vi "get parameters.vi"(8 "error in (no error)":errorcluster, 11 "Task.lvclass in":refnum<class "Task.lvclass">) -> (0 "error out":errorcluster, 2 "parameters":T1, 3 "Task.lvclass out":refnum<class "Task.lvclass">)   [LabVIEW 2020, in "Tasks.lvlib" / "Task.lvclass"]
uses:
  Task.lvclass
  parameters.ctl
  Task.lvclass/Task.ctl
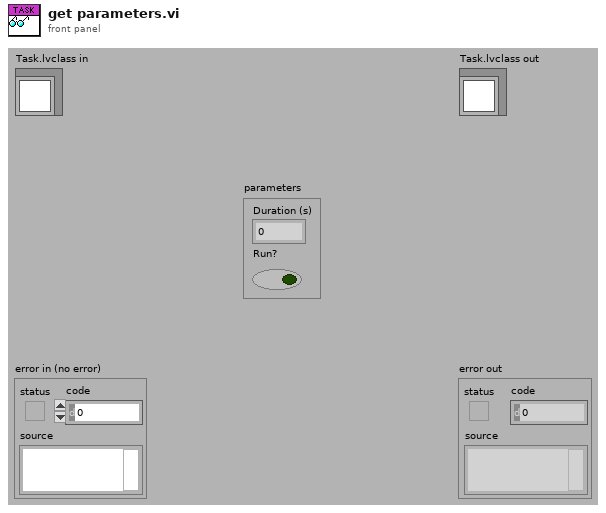
[diagram p1: front panel]
types:
  T1 = typedef "Tasks.lvlib/Task.lvclass/parameters.ctl" = cluster{"Duration (s)":dbl, "Run?":bool}
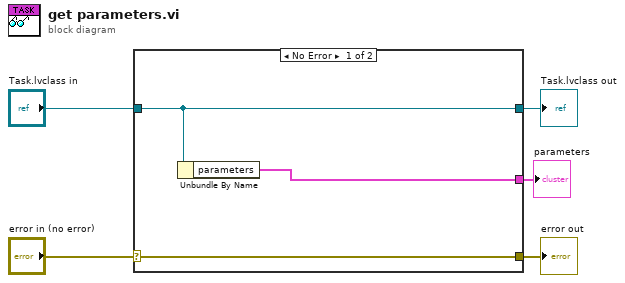
[diagram p0: block diagram]
diagram:
  n1 = case shown="No Error" "error in (no error)" {
    selector: "error in (no error)" -> [w8 w9]
    tunnel: [w8 w9] -> w4
    tunnel: [w7 w10] -> w2
    tunnel: "Task.lvclass in" -> [w7 w10]
    tunnel: [w6 _] -> w1
    frame No Error {
      n2 = Unbundle By Name(w7) -> ("parameters"=w6:T1)
    }
    frame Error {
    }
  }
  "error out" <- w4
  "Task.lvclass out" <- w2
  "parameters" <- w1
